vi "SynchIRQ.vi"(0 "WaveformAddressSpace":refnum<class "WaveformAddressSpace.lvclass">) -> ()   [LabVIEW 2015]
uses:
  <vilib>/rvi/DataTransferAndStorage/Container/XNode/niFpgaContainer.xnode
  <vilib>/rvi/DataTransferAndStorage/Register/Emulation/niFpgaRegisterEmulationRefIn.vi
  WaveformAddressSpace.lvclass
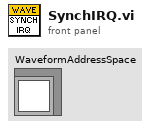
[diagram p1: front panel]
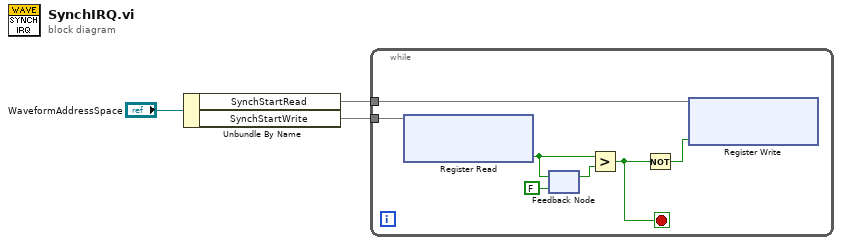
[diagram p0: block diagram]
diagram:
  n1 = Unbundle By Name("WaveformAddressSpace") -> ("SynchStartRead"=w2, "SynchStartWrite"=w1)
  n2 = while {
    tunnel: w2 -> [w5]
    tunnel: w1 -> [w10]
    stop <- w6 stop-if-true
    n3 = xnode "Register Read"("Register In"=w10) -> ("Data"=w7:bool)  [unwired: 1 out]
    n4 = feedback-in #1(w7) -> ()
    n5 = feedback #1(FALSE ("Data")) -> (w8:bool)
    n6 = Greater?(x=w7, y=w8) -> (0:w6:bool)
    n7 = Not(x=w6) -> (.not. x?=w4:bool)
    n8 = xnode "Register Write"("Data"=w4, "Register In"=w5) -> ()  [unwired: 1 out]
  }
